vi "Generate Display Element DVR.vi"(8 "Error In":errorcluster, 11 "Display Element In":refnum<class "Display Element.lvclass">) -> (0 "Error Out":errorcluster, 3 "Display Element Out":refnum<class "Display Element.lvclass">)   [LabVIEW 2019, in "Display Element.lvclass"]
uses:
  Display Element.lvclass
  Controls/Data.ctl
  Public/Controls/Vector.ctl
  Display Element.lvclass/Display Element.ctl
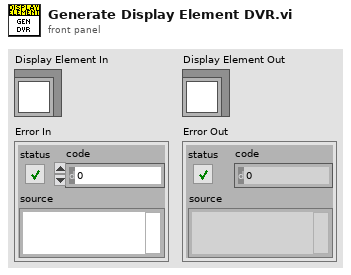
[diagram p1: front panel]
types:
  T1 = typedef "Display Element.lvclass/Data.ctl" = cluster{"Color":u32, "Layer":u32, "Tag":string, "Position":T2, "Force":T2, "Delete If Outside Bounds":bool}
  T2 = typedef "Display Element.lvclass/Vector.ctl" = cluster{"X":i32, "Y":i32}
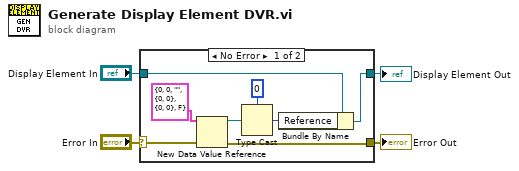
[diagram p0: block diagram]
diagram:
  n1 = case shown="No Error" "Error In" {
    selector: "Error In" -> [w12 w14]
    tunnel: "Display Element In" -> [w9 w13]
    tunnel: [w6 w14] -> w1
    tunnel: [w7 w13] -> w3
    frame No Error {
      n2 = New Data Value Reference(data value=T1 {"Color"=0, "Layer"=0, "Tag"="", "Position"={"X"=0, "Y"=0}, "Force"={"X"=0, "Y"=0}, "Delete If Outside Bounds"=FALSE} ("Data"), error in=w12) -> (data value reference=w10:refnum<data-value>, error out=w6:errorcluster)
      n3 = Type Cast(type=u64 0, x=w10) -> (*(type *) &x=w8:u64)
      n4 = Bundle By Name(cluster=w9, "Reference"=w8) -> (w7:refnum<class "Display Element.lvclass">)
    }
    frame Error {
    }
  }
  "Display Element Out" <- w3
  "Error Out" <- w1
